vi "J-KEM_subVI.vi"(7 "Control temp":bool, 10 "Address in":T1, 11 "J-KEM on?":bool) -> (0 "Temp (C)":dbl format="%#_6f", 1 "String data out":string, 3 "Address out":T1)   [LabVIEW 2014]
panel:
  out "read buffer":string
  in  "Set temp (C)":i32
  out "concatenated string":string
  in  "Stop Button":bool
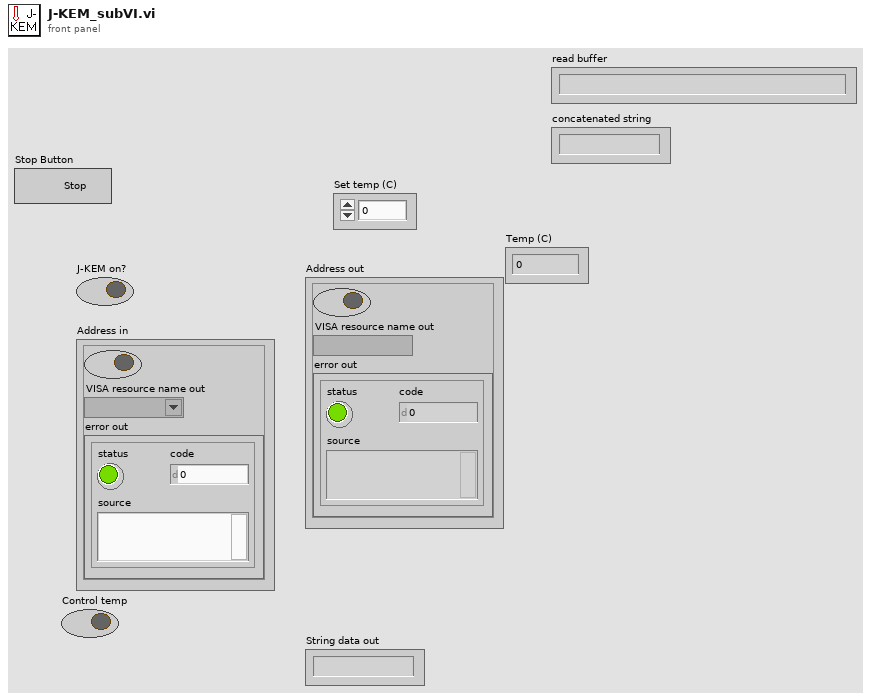
[diagram p1: front panel]
types:
  T1 = cluster{"Boolean":bool, "VISA resource name out":refnum<visa-resource-name>, "error out":errorcluster}
  T2 = cluster{bool, "VISA resource name out":refnum<visa-resource-name>, "error out":errorcluster}
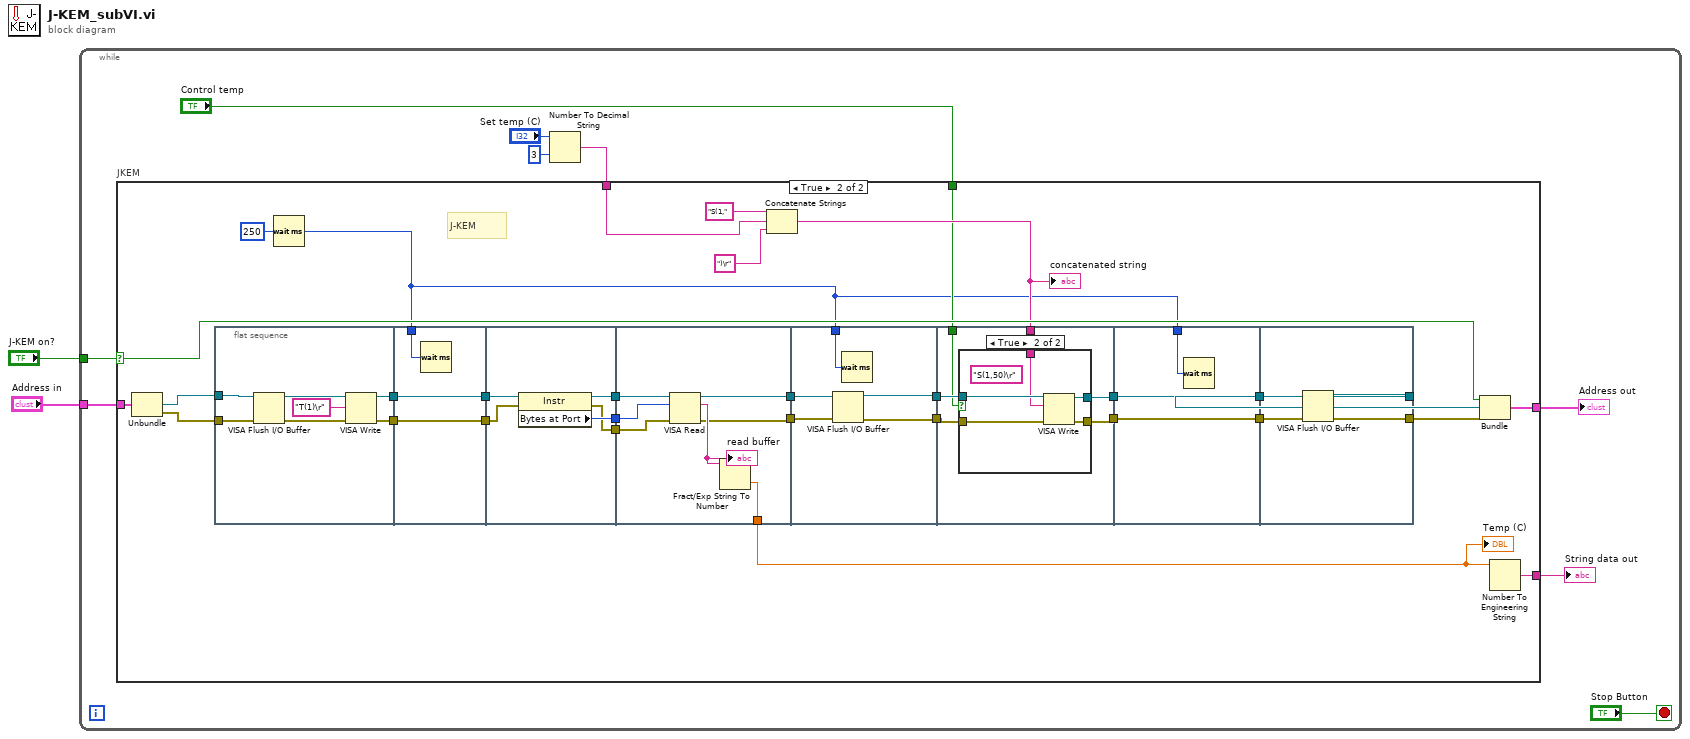
[diagram p0: block diagram]
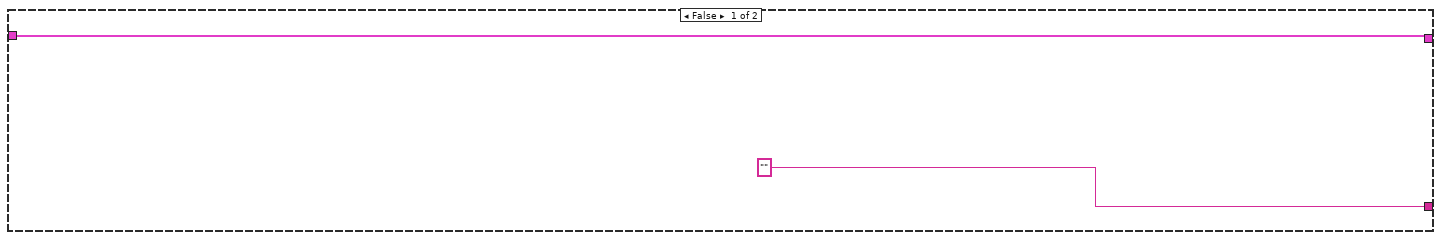
[diagram p2: hidden frame]
diagram:
  n1 = while {
    tunnel: "J-KEM on?" -> [w11]
    tunnel: "Address in" -> [w8]
    stop <- "Stop Button" stop-if-true
    n2 = Number To Decimal String(number="Set temp (C)", width (-)=i16 3 ("precision (6)")) -> (decimal integer string=w7:string)
    n3 = case "JKEM" shown="True" w11 {
      selector: w11 -> [_ w38]
      tunnel: w8 -> [w13 w42]
      tunnel: [w13 w40] -> w9
      tunnel: ["" w39] -> w10
      tunnel: w7 -> [_ w22]
      tunnel: "Control temp" -> [_ w20]
      frame False {
      }
      frame True {
        w14 = u32 250 ("milliseconds to wait")
        # "J-KEM"
        n4 = Unbundle(w42) -> ("VISA resource name out"=w41:refnum<visa-resource-name>, "error out"=w37:errorcluster)  [unwired: 1 out]
        n5 = flat-sequence {
          tunnel: w41 -> [w48]
          tunnel: w37 -> [w46]
          tunnel: [w50] -> w35
          tunnel: [w49] -> w34
          tunnel: w14 -> [w53]
          tunnel: [w52] -> w33
          tunnel: w35 -> [w52]
          tunnel: w34 -> [w51]
          tunnel: [w51] -> w32
          tunnel: w33 -> [w58]
          tunnel: w32 -> [w57]
          tunnel: [w56] -> w31
          tunnel: [w55] -> w30
          tunnel: [w54] -> w29
          tunnel: w31 -> [w65]
          tunnel: w30 -> [w64]
          tunnel: w29 -> [w63]
          tunnel: [w59] -> w36
          tunnel: [w60] -> w28
          tunnel: [w61] -> w27
          tunnel: w28 -> [w67]
          tunnel: w27 -> [w69]
          tunnel: [w66] -> w26
          tunnel: [w68] -> w25
          tunnel: w14 -> [w70]
          tunnel: w26 -> [w75]
          tunnel: w25 -> [w76]
          tunnel: w21 -> [w72]
          tunnel: w20 -> [w71]
          tunnel: [w73] -> w19
          tunnel: [w74] -> w18
          tunnel: w19 -> [w85]
          tunnel: w18 -> [w86]
          tunnel: [w85] -> w16
          tunnel: [w86] -> w15
          tunnel: w14 -> [w84]
          tunnel: [w89] -> w43
          tunnel: [w87] -> w17
          tunnel: w16 -> [w88]
          tunnel: w15 -> [w90]
          frame #0 {
            n6 = VISA Flush I/O Buffer(VISA resource name=w48, error in (no error)=w46) -> (VISA resource name out=w47:refnum<visa-resource-name>, error out=w45:errorcluster)  [unwired: 1 in]
            n7 = VISA Write(VISA resource name=w47, write buffer="T(1)\r", error in (no error)=w45) -> (VISA resource name out=w50:refnum<visa-resource-name>, error out=w49:errorcluster)  [unwired: 1 out]
          }
          frame #1 {
            n8 = Wait (ms)(milliseconds to wait=w53) -> ()  [unwired: 1 out]
          }
          frame #2 {
            n9 = property class="Instr"(reference=w58, error in=w57) -> (reference out=w56:refnum<visa-resource-name>, error out=w54:errorcluster, "Bytes at Port"=w55:u32)
          }
          frame #3 {
            n10 = VISA Read(VISA resource name=w65, byte count=w64, error in (no error)=w63) -> (VISA resource name out=w61:refnum<visa-resource-name>, read buffer=w62:string, error out=w60:errorcluster)  [unwired: 1 out]
            "read buffer" <- w62
            n11 = Fract/Exp String To Number(string=w62) -> (number=w59:dbl)  [unwired: 3 in, 1 out]
          }
          frame #4 {
            n12 = VISA Flush I/O Buffer(VISA resource name=w69, error in (no error)=w67) -> (VISA resource name out=w68:refnum<visa-resource-name>, error out=w66:errorcluster)  [unwired: 1 in]
            n13 = Wait (ms)(milliseconds to wait=w70) -> ()  [unwired: 1 out]
          }
          frame #5 {
            n14 = case shown="True" w71 {
              tunnel: w76 -> [w78 w83]
              tunnel: w75 -> [w77 w82]
              tunnel: [w78 w81] -> w74
              tunnel: [w77 w80] -> w73
              tunnel: w72 -> [_ w79]
              frame False {
              }
              frame True {
                (unwired) "S(1,50)\r" ("write buffer")
                n15 = VISA Write(VISA resource name=w83, write buffer=w79, error in (no error)=w82) -> (VISA resource name out=w81:refnum<visa-resource-name>, error out=w80:errorcluster)  [unwired: 1 out]
              }
            }
          }
          frame #6 {
            n16 = Wait (ms)(milliseconds to wait=w84) -> ()  [unwired: 1 out]
          }
          frame #7 {
            n17 = VISA Flush I/O Buffer(VISA resource name=w90, error in (no error)=w88) -> (VISA resource name out=w89:refnum<visa-resource-name>, error out=w87:errorcluster)  [unwired: 1 in]
          }
        }
        n18 = Wait (ms)(milliseconds to wait=w14) -> ()  [unwired: 1 out]
        n19 = Concatenate Strings("S(1," ("write buffer"), w22, ")\r" ("write buffer")) -> (w21:string)
        "concatenated string" <- w21
        n20 = Bundle(w38, "VISA resource name out"=w43, "error out"=w17) -> (w40:T2)  [unwired: 1 in]
        n21 = Number To Engineering String(4:w36) -> (0:w39:string)  [unwired: 3 in]
        "Temp (C)" <- w36
      }
    }
    "String data out" <- w10
    "Address out" <- w9
  }
